vi "GetParam.vi"(8 "error in (no error)":errorcluster caption="entrée d'erreur (pas d'erreur)", 11 "StratifiedShuffleSplit.lvclass":refnum<class "StratifiedShuffleSplit.lvclass">) -> (0 "error out":errorcluster caption="sortie d'erreur", 2 "StratifiedShuffleSplit":T1={"n_splits"=10, "test_size"="None", "train_size"="None", "random_state"=-1} {"random_state" min=-1}, 3 "StratifiedShuffleSplit.lvclass":refnum<class "StratifiedShuffleSplit.lvclass">)   [LabVIEW 2020, in "StratifiedShuffleSplit.lvclass"]
doc: "Get Parameters"
uses:
  StratifiedShuffleSplit.lvclass
  StratifiedShuffleSplit.lvclass/StratifiedShuffleSplit.ctl
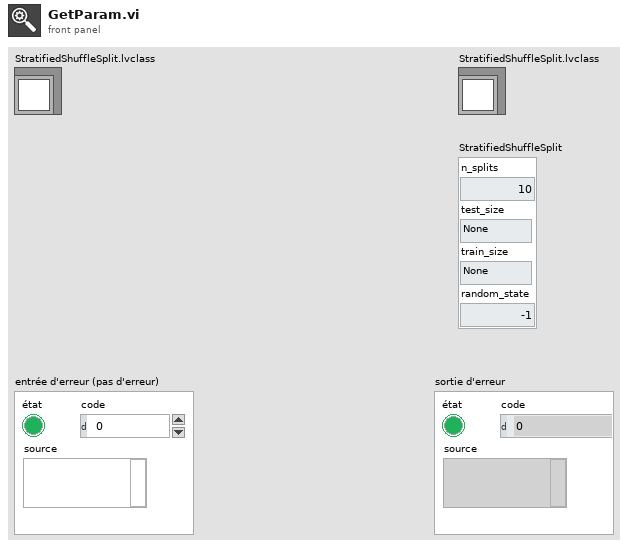
[diagram p1: front panel]
types:
  T1 = cluster{"n_splits":i32, "test_size":string, "train_size":string, "random_state":i32}
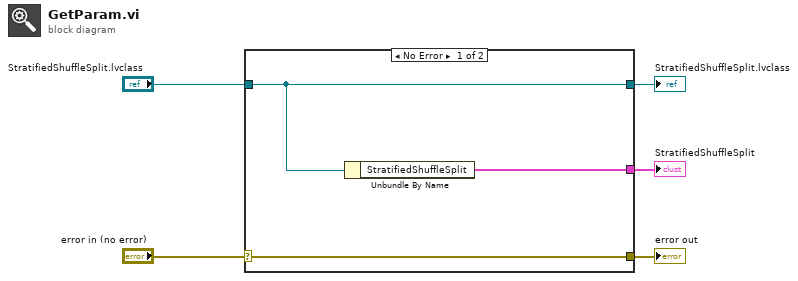
[diagram p0: block diagram]
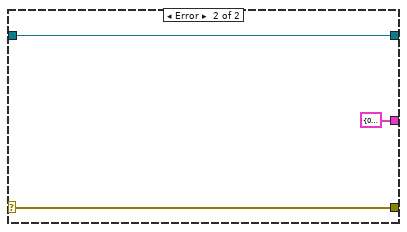
[diagram p2: hidden frame]
diagram:
  n1 = case shown="No Error" "error in (no error)" {
    selector: "error in (no error)" -> [w8 w10]
    tunnel: [w8 w10] -> w4
    tunnel: [w7 w11] -> w2
    tunnel: "StratifiedShuffleSplit.lvclass" -> [w7 w11]
    tunnel: [w6 T1 {"n_splits"=0, "test_size"="", "train_size"="", "random_state"=0} ("StratifiedShuffleSplit")] -> w1
    frame No Error {
      n2 = Unbundle By Name(w7) -> ("StratifiedShuffleSplit"=w6:T1)
    }
    frame Error {
    }
  }
  "error out" <- w4
  "StratifiedShuffleSplit.lvclass" <- w2
  "StratifiedShuffleSplit" <- w1
